vi "Queue.vi"(1 "Timeout":i32=-1, 2 "Mode":u16(ring) items=["Push", "Pop"], 3 "Value In":variant, 4 "Name":string) -> (0 "Value Out":variant)   [LabVIEW 2014]
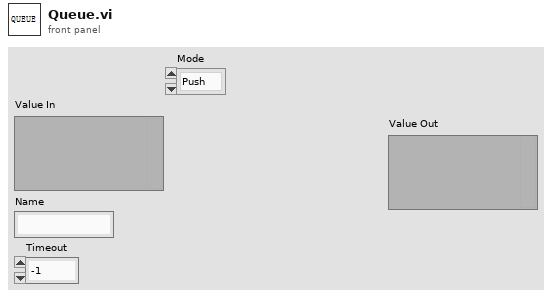
[diagram p1: front panel]
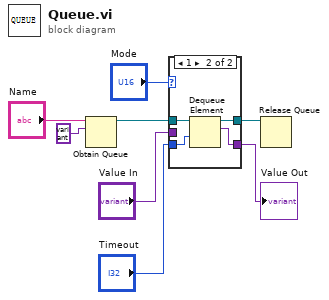
[diagram p0: block diagram]
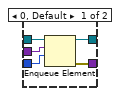
[diagram p2: hidden frame]
diagram:
  n1 = Obtain Queue(name (unnamed)="Name", element data type=variant) -> (queue out=w5:refnum<queue>)  [unwired: 3 in, 2 out]
  n2 = case shown="1" "Mode" {
    tunnel: w5 -> [w13 w17]
    tunnel: "Value In" -> [w12 _]
    tunnel: [w11 w16] -> w4
    tunnel: [w10 w15] -> w3
    tunnel: "Timeout" -> [w9 w14]
    frame 0, Default {
      n3 = Enqueue Element(queue=w13, element=w12, timeout in ms (-1)=w9) -> (queue out=w11:refnum<queue>, error out=w10:errorcluster)  [unwired: 1 in, 1 out]
    }
    frame 1 {
      n4 = Dequeue Element(queue=w17, timeout in ms (-1)=w14) -> (queue out=w16:refnum<queue>, element=w15:variant)  [unwired: 1 in, 2 out]
    }
  }
  "Value Out" <- w3
  n5 = Release Queue(queue=w4) -> ()  [unwired: 2 in, 3 out]
